vi "_Update XML Method.vi"(6 "SourceProperties":T1[](array[typedef]) {"Source Type" items=["APCI 1", "APCI 2", "ESI 1", "ESI 2"]}, 8 "DOM document":refnum<k20>) -> (0 "error out":errorcluster, 3 "DOM document out":refnum<k20>)   [LabVIEW 2012]
uses:
  _Source Properties.ctl
  _XML Source Type.ctl
  <vilib>/xml/Close Reference(Node).vi
  <resource>/objmgr/DOMUserDefRef.rc
  <vilib>/xml/NI_XML.lvlib
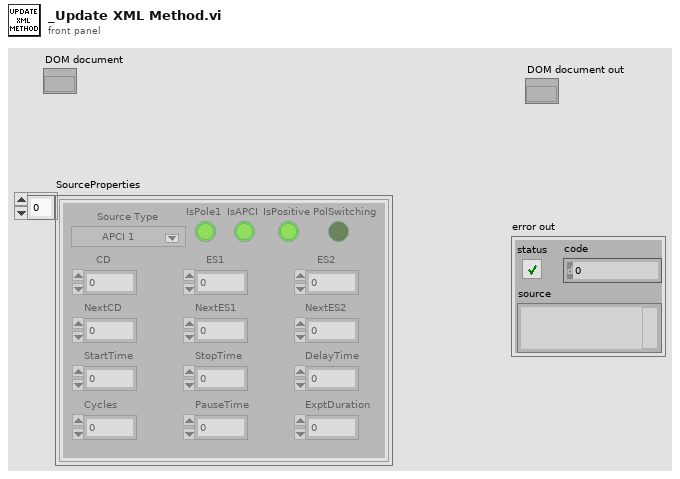
[diagram p1: front panel]
types:
  T1 = typedef "_Source Properties.ctl" = cluster{"Source Type":T2, "IsPole1":bool, "IsAPCI":bool, "IsPositive":bool, "CD":dbl, "ES1":dbl, "ES2":dbl, "NextCD":dbl, "NextES1":dbl, "NextES2":dbl, "PolSwitching":bool, "StartTime":dbl, "StopTime":dbl, "DelayTime":dbl, "Cycles":i32, "PauseTime":dbl, "ExptDuration":dbl}
  T2 = typedef "_XML Source Type.ctl" = u16
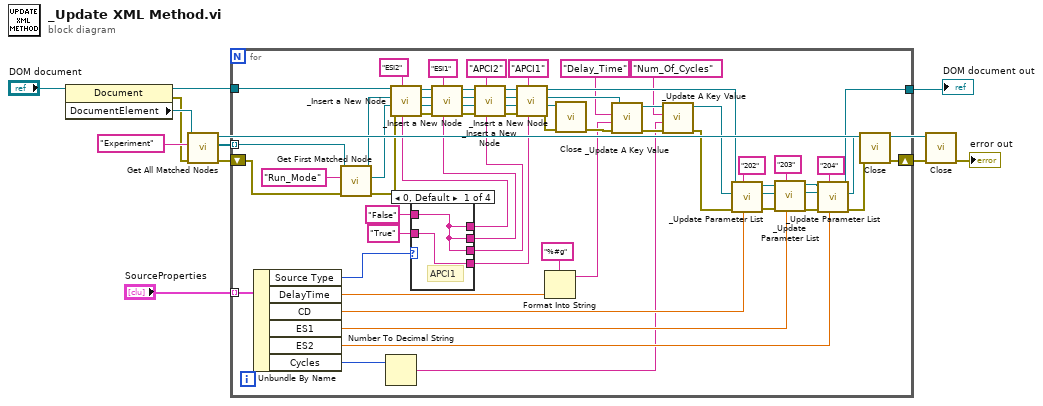
[diagram p0: block diagram]
diagram:
  n1 = property on="Property Node" class="Document"(reference="DOM document") -> (reference out=w6:refnum<k20>, error out=w8:errorcluster, "DocumentElement"=w9:refnum<k20>)  [unwired: 1 in]
  n2 = call <vilib>:"Get All Matched Nodes.vi"("error in (no error)"=w8, "XPath expression"="Experiment", "node in"=w9) -> ("error out"=w5:errorcluster, "node result array"=w7:refnum<k20>[], "node out"=w4:refnum<k20>)  [unwired: 6 in]
  n3 = for {
    tunnel: w7 -> [w74] mode=indexing
    tunnel: w6 -> [w72]
    shift-right: [w44] -> w3
    shift-left: w5 -> [w73]
    tunnel: [w31] -> w2
    tunnel: "SourceProperties" -> [w30] mode=indexing
    n4 = Unbundle By Name(w30) -> ("Source Type"=w26:T2, "DelayTime"=w22:dbl, "CD"=w29:dbl, "ES1"=w28:dbl, "ES2"=w27:dbl, "Cycles"=w19:i32)
    n5 = call <vilib>:"Get First Matched Node.vi"("error in (no error)"=w73, "XPath expression"="Run_Mode", "node in"=w74) -> ("error out"=w68:errorcluster, "node result"=w70:refnum<k20>, "node out"=w69:refnum<k20>)  [unwired: 6 in]
    n6 = Number To Decimal String(number=w19) -> (decimal integer string=w15:string)  [unwired: 1 in]
    n7 = case shown="0, Default" w26 {
      tunnel: [w77 w79 w81 w82] -> w65
      tunnel: [w77 w79 w80 w83] -> w62
      tunnel: [w77 w78 w81 w83] -> w53
      tunnel: [w76 w79 w81 w83] -> w50
      tunnel: "False" -> [w77 w79 w81 w83]
      tunnel: "True" -> [w76 w78 w80 w82]
      frame 0, Default {
        # "APCI1"
      }
      frame 1 {
        # "APCI2"
      }
      frame 2 {
        # "ESI1"
      }
      frame 3 {
        # "ESI2"
      }
    }
    n8 = call "_Insert a New Node.vi"("Data"=w65, "Tag Name"="ESI2", "error in (no error)"=w68, "Reference Child"=w70, "Experiment Node"=w69, "DOM Document"=w72) -> ("error out"=w64:errorcluster, "Reference Child out"=w59:refnum<k20>, "Experiment Node out"=w60:refnum<k20>, "DOM Document out"=w61:refnum<k20>)  [unwired: 2 in]
    n9 = call "_Insert a New Node.vi"("Data"=w62, "Tag Name"="ESI1", "error in (no error)"=w64, "Reference Child"=w59, "Experiment Node"=w60, "DOM Document"=w61) -> ("error out"=w57:errorcluster, "Reference Child out"=w54:refnum<k20>, "Experiment Node out"=w55:refnum<k20>, "DOM Document out"=w56:refnum<k20>)  [unwired: 2 in]
    n10 = call "_Insert a New Node.vi"("Data"=w53, "Tag Name"="APCI2", "error in (no error)"=w57, "Reference Child"=w54, "Experiment Node"=w55, "DOM Document"=w56) -> ("error out"=w51:errorcluster, "Reference Child out"=w47:refnum<k20>, "Experiment Node out"=w48:refnum<k20>, "DOM Document out"=w49:refnum<k20>)  [unwired: 2 in]
    n11 = call "_Insert a New Node.vi"("Data"=w50, "Tag Name"="APCI1", "error in (no error)"=w51, "Reference Child"=w47, "Experiment Node"=w48, "DOM Document"=w49) -> ("error out"=w46:errorcluster, "Reference Child out"=w45:refnum<k20>, "Experiment Node out"=w25:refnum<k20>, "DOM Document out"=w43:refnum<k20>)  [unwired: 2 in]
    n12 = Format Into String(format string="%#g", w22) -> (resulting string=w21:string)  [unwired: 2 in, 1 out]
    n13 = call-poly <vilib>:"Close.vi"("error in (no error)"=w46, "node"=w45) -> ("error out"=w24:errorcluster)  [unwired: 7 in]
    n14 = call "_Update A Key Value.vi"("error in (no error)"=w24, "Value"=w21, "Key"="Delay_Time", "node in"=w25) -> ("error out"=w18:errorcluster, "node out"=w17:refnum<k20>)  [unwired: 2 in]
    n15 = call "_Update A Key Value.vi"("error in (no error)"=w18, "Value"=w15, "Key"="Num_Of_Cycles", "node in"=w17) -> ("error out"=w13:errorcluster, "node out"=w14:refnum<k20>)  [unwired: 2 in]
    n16 = call "_Update Parameter List.vi"("Data"=w29, "Channel ID"="202" ("Tag Name"), "error in (no error)"=w13, "Experiment Node"=w14, "DOM Document"=w43) -> ("error out"=w40:errorcluster, "Experiment Node out"=w38:refnum<k20>, "DOM Document out"=w39:refnum<k20>)  [unwired: 4 in]
    n17 = call "_Update Parameter List.vi"("Data"=w28, "Channel ID"="203" ("Tag Name"), "error in (no error)"=w40, "Experiment Node"=w38, "DOM Document"=w39) -> ("error out"=w36:errorcluster, "Experiment Node out"=w34:refnum<k20>, "DOM Document out"=w35:refnum<k20>)  [unwired: 4 in]
    n18 = call "_Update Parameter List.vi"("Data"=w27, "Channel ID"="204" ("Tag Name"), "error in (no error)"=w36, "Experiment Node"=w34, "DOM Document"=w35) -> ("error out"=w33:errorcluster, "Experiment Node out"=w32:refnum<k20>, "DOM Document out"=w31:refnum<k20>)  [unwired: 4 in]
    n19 = call-poly <vilib>:"Close.vi"("error in (no error)"=w33, "node"=w32) -> ("error out"=w44:errorcluster)  [unwired: 7 in]
  }
  "DOM document out" <- w2
  n20 = call-poly <vilib>:"Close.vi"("error in (no error)"=w3, "node"=w4) -> ("error out"=→"error out":errorcluster)  [unwired: 7 in]
